vi "Sine Sweep Signal.vi"(0 "reference in":refnum<class "GSwFormDSP.lvclass">, 5 "error in (no error)":errorcluster) -> (14 "reference in":refnum<class "GSwFormDSP.lvclass">, 19 "error out":errorcluster)   [LabVIEW 2020, in "GSwFormDSP.lvclass"]
uses:
  GSwFormDSP.lvclass
panel:
  out "FS":dbl
  in  "Done":bool
  in  "Duration (s)":dbl=10.0 min=1.0 max=3600.0 step=0.1 format="%.1f"
  in  "User Input Fs":T1(ring)=enum."44100 Hz" caption="Sampling Rate"
  in  "Freq start (Hz)":dbl=100.0 min=0.0 max=22050.0 step=1.0 format="%.2f"
  in  "Freq end (Hz)":dbl=10000.0 min=0.0 max=22050.0 step=1.0 format="%.2f"
  in  "Amplitude":dbl=1.0 format="%.2f"
  in  "Signal Name":string="unknown"
  in  "Signal Unit":string="unknown"
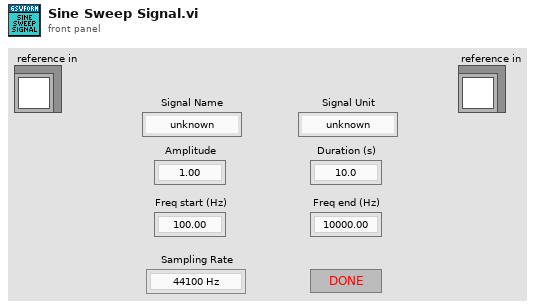
[diagram p1: front panel]
types:
  T1 = enum16{"256 Hz", "512 Hz", "1024 Hz", "2048 Hz", "4096 Hz", "8192 Hz", "11025 Hz", "16384 Hz", "22050 Hz", "32768 Hz", "44100 Hz"}
  T2 = enum16{"Replace Current Signals", "Append to Current Signals"}
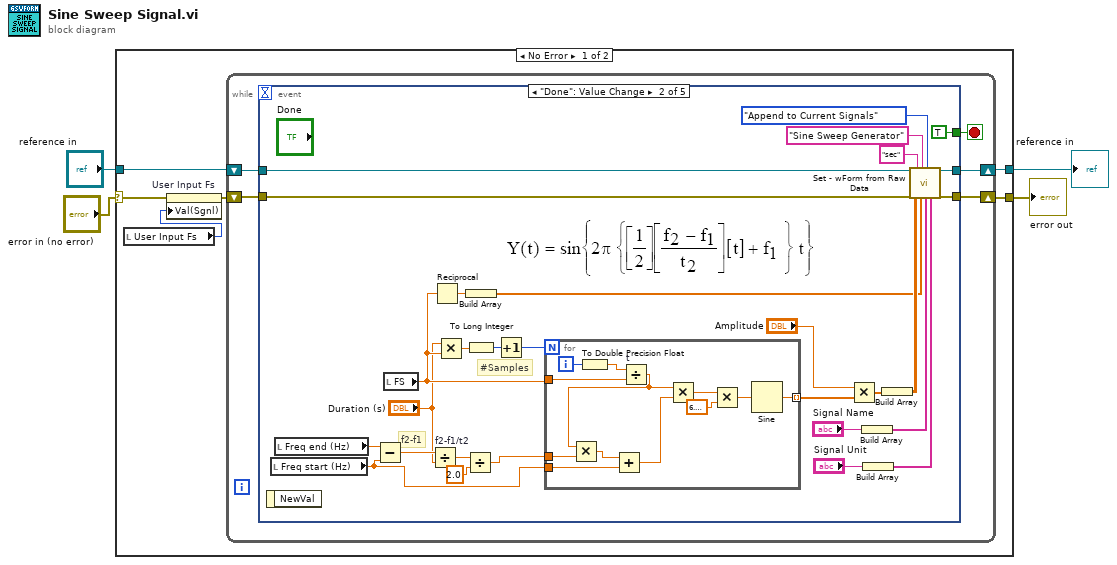
[diagram p0: block diagram]
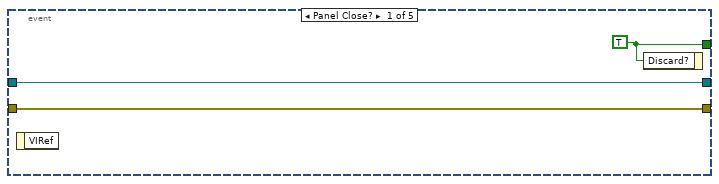
[diagram p2: hidden frame]
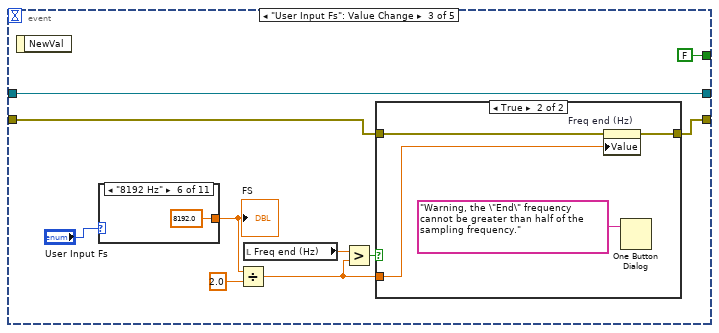
[diagram p3: hidden frame]
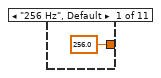
[diagram p5: hidden frame]
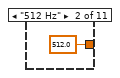
[diagram p6: hidden frame]
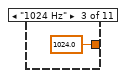
[diagram p7: hidden frame]
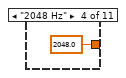
[diagram p8: hidden frame]
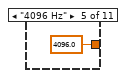
[diagram p9: hidden frame]
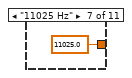
[diagram p10: hidden frame]
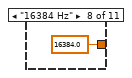
[diagram p11: hidden frame]
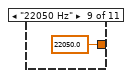
[diagram p12: hidden frame]
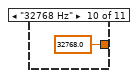
[diagram p13: hidden frame]
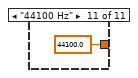
[diagram p14: hidden frame]
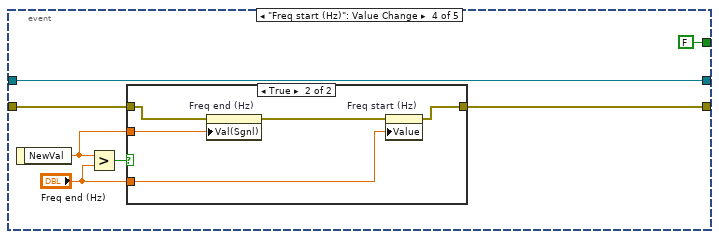
[diagram p15: hidden frame]
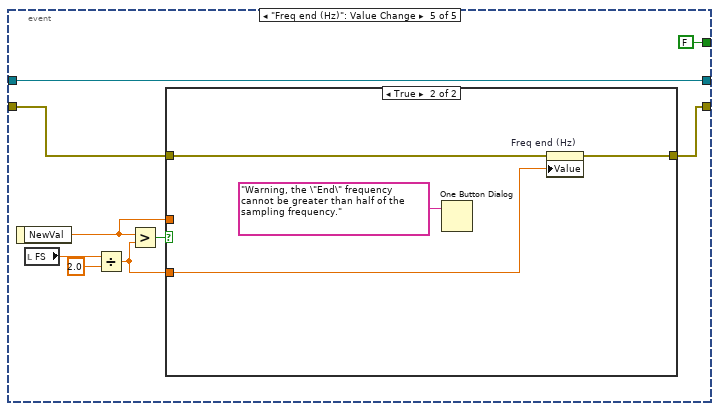
[diagram p17: hidden frame]
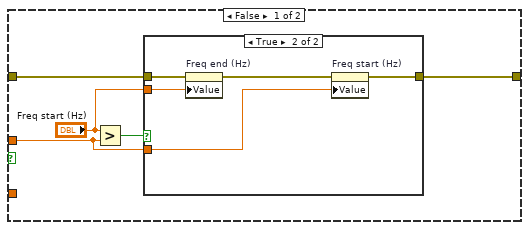
[diagram p18: hidden frame]
diagram:
  n1 = case shown="No Error" "error in (no error)" {
    selector: "error in (no error)" -> [w5 w124]
    tunnel: [w8 w124] -> w3
    tunnel: [w9 w123] -> w1
    tunnel: "reference in" -> [w10 w123]
    frame No Error {
      n2 = local read "User Input Fs"() -> (w6:T1)
      n3 = property on="User Input Fs" class="Enum (strict)"(error in=w5, "Val(Sgnl)"=w6) -> (error out=w7:errorcluster)  [unwired: 1 in, 1 out]
      n4 = while {
        shift-right: [w13] -> w9
        shift-left: w10 -> [w14]
        shift-right: [w12] -> w8
        shift-left: w7 -> [w11]
        stop <- w15 stop-if-true
        n5 = event shown="[1] \"Done\": Value Change" {
          selector: _ -> [_ _ _ _ _]
          dyn-events: _ -> [_ _ _ _ _]
          timeout: _ -> [_ _ _ _ _]
          tunnel: [w18 TRUE ("Discard?") FALSE ("Discard?") FALSE ("Discard?") FALSE ("Discard?")] -> w15
          tunnel: w14 -> [w17 w24 w67 w91 w106]
          tunnel: [w17 w23 w67 w91 w106] -> w13
          tunnel: [w16 w22 w61 w86 w102] -> w12
          tunnel: w11 -> [w16 w21 w62 w89 w103]
          event Panel Close? {
            w18 = TRUE ("Discard?")
            n6 = event-data() -> ()  [unwired: 1 in, 1 out]
            n7 = event-data("Discard?"=w18) -> ()  [unwired: 1 in, 1 out]
          }
          event "Done": Value Change {
            # "#Samples"
            # "f2-f1"
            n8 = event-data() -> ()  [unwired: 1 in, 1 out]
            n9 = local read "Freq start (Hz)"() -> (w28:dbl)
            n10 = local read "Freq end (Hz)"() -> (w29:dbl)
            n11 = Subtract(x=w29, y=w28) -> (x-y=w45:dbl)
            n12 = local read "FS"() -> (w30:dbl)
            n13 = Divide "f2-f1/t2"(x=w45, y="Duration (s)") -> (x/y=w42:dbl)
            n14 = Reciprocal(x=w30) -> (1/x=w38:dbl)
            n15 = Multiply(x="Duration (s)", y=w30) -> (x*y=w46:dbl)
            n16 = Divide(x=w42, y=2.0) -> (x/y=w40:dbl)
            n17 = Build Array(w38) -> (w34:dbl[])
            n18 = To Long Integer(number=w46) -> (32bit integer=w41:i32)
            n19 = Increment(x=w41) -> (x+1=w43:i32)
            n20 = for {
              N: w43 -> [_]
              tunnel: [w57] -> w44 mode=indexing
              tunnel: w40 -> [w56]
              tunnel: w28 -> [w54]
              tunnel: w30 -> [w53]
              i -> [w50]
              n21 = To Double Precision Float(number=w50) -> (double precision float=w49:dbl)
              n22 = Divide "t"(x=w49, y=w53) -> (x/y=w48:dbl)
              n23 = Multiply(x=w48, y=w56) -> (x*y=w55:dbl)
              n24 = Add(x=w55, y=w54) -> (x+y=w51:dbl)
              n25 = Multiply(x=w48, y=w51) -> (x*y=w52:dbl)
              n26 = Multiply(x=w52, y=6.283185307179586) -> (x*y=w59:dbl)
              n27 = Sine(x=w59) -> (sin(x)=w57:dbl)
            }
            n28 = Multiply(x="Amplitude", y=w44) -> (x*y=w27:dbl[])
            n29 = Build Array("Signal Name") -> (w33:string[])
            n30 = Build Array("Signal Unit") -> (w32:string[])
            n31 = Build Array(w27) -> (w35:dbl[][])
            n32 = call "Set - wForm from Raw Data.vi"("reference in"=w24, "error in (no error)"=w21, "X Unit"="sec", "Y Data (Row matrix)"=w35, "Data Origin"="Sine Sweep Generator", "dTs"=w34, "Signal Set"=T2."Append to Current Signals", "Signals Name"=w33, "Signals Unit"=w32) -> ("reference in"=w23:refnum<class "GSwFormDSP.lvclass">, "error out"=w22:errorcluster)  [unwired: 9 in]
          }
          event "User Input Fs": Value Change {
            n33 = event-data() -> ()  [unwired: 1 in, 1 out]
            n34 = case shown="\"8192 Hz\"" "User Input Fs" {
              tunnel: [256.0 512.0 1024.0 2048.0 4096.0 8192.0 11025.0 16384.0 22050.0 32768.0 44100.0] -> w65
              frame "256 Hz", Default {
              }
              frame "512 Hz" {
              }
              frame "1024 Hz" {
              }
              frame "2048 Hz" {
              }
              frame "4096 Hz" {
              }
              frame "8192 Hz" {
              }
              frame "11025 Hz" {
              }
              frame "16384 Hz" {
              }
              frame "22050 Hz" {
              }
              frame "32768 Hz" {
              }
              frame "44100 Hz" {
              }
            }
            "FS" <- w65
            n35 = Divide(x=w65, y=2.0) -> (x/y=w60:dbl)
            n36 = local read "Freq end (Hz)"() -> (w64:dbl)
            n37 = Greater?(x=w64, y=w60) -> (0:w63:bool)
            n38 = case shown="True" w63 {
              tunnel: w62 -> [w70 w73]
              tunnel: [w70 w72] -> w61
              tunnel: w60 -> [_ w71]
              frame False {
              }
              frame True {
                n39 = property on="Freq end (Hz)" class="DigNum (strict)"(error in=w73, "Value"=w71) -> (error out=w72:errorcluster)  [unwired: 1 in, 1 out]
                n40 = One Button Dialog(message="Warning, the \"End\" frequency cannot be greater than half of the sampling frequency.") -> ()  [unwired: 1 in, 1 out]
              }
            }
          }
          event "Freq start (Hz)": Value Change {
            n41 = event-data() -> ("NewVal"=w88:dbl)  [unwired: 1 in]
            n42 = Greater?(x=w88, y="Freq end (Hz)") -> (0:w90:bool)
            n43 = case shown="True" w90 {
              tunnel: w89 -> [w93 w98]
              tunnel: w88 -> [_ w97]
              tunnel: "Freq end (Hz)" -> [_ w96]
              tunnel: [w93 w94] -> w86
              frame False {
              }
              frame True {
                n44 = property on="Freq end (Hz)" class="DigNum (strict)"(error in=w98, "Val(Sgnl)"=w97) -> (error out=w95:errorcluster)  [unwired: 1 in, 1 out]
                n45 = property on="Freq start (Hz)" class="DigNum (strict)"(error in=w95, "Value"=w96) -> (error out=w94:errorcluster)  [unwired: 1 in, 1 out]
              }
            }
          }
          event "Freq end (Hz)": Value Change {
            n46 = event-data() -> ("NewVal"=w104:dbl)  [unwired: 1 in]
            n47 = local read "FS"() -> (w100:dbl)
            n48 = Divide(x=w100, y=2.0) -> (x/y=w99:dbl)
            n49 = Greater?(x=w104, y=w99) -> (0:w105:bool)
            n50 = case shown="True" w105 {
              tunnel: w104 -> [w110 _]
              tunnel: w103 -> [w109 w121]
              tunnel: [w108 w120] -> w102
              tunnel: w99 -> [_ w119]
              frame False {
                n51 = Greater?(x="Freq start (Hz)", y=w110) -> (0:w112:bool)
                n52 = case shown="True" w112 {
                  tunnel: "Freq start (Hz)" -> [_ w118]
                  tunnel: w110 -> [_ w117]
                  tunnel: w109 -> [w113 w115]
                  tunnel: [w113 w114] -> w108
                  frame False {
                  }
                  frame True {
                    n53 = property on="Freq end (Hz)" class="DigNum (strict)"(error in=w115, "Value"=w118) -> (error out=w116:errorcluster)  [unwired: 1 in, 1 out]
                    n54 = property on="Freq start (Hz)" class="DigNum (strict)"(error in=w116, "Value"=w117) -> (error out=w114:errorcluster)  [unwired: 1 in, 1 out]
                  }
                }
              }
              frame True {
                n55 = One Button Dialog(message="Warning, the \"End\" frequency cannot be greater than half of the sampling frequency.") -> ()  [unwired: 1 in, 1 out]
                n56 = property on="Freq end (Hz)" class="DigNum (strict)"(error in=w121, "Value"=w119) -> (error out=w120:errorcluster)  [unwired: 1 in, 1 out]
              }
            }
          }
        }
      }
    }
    frame Error {
    }
  }
  "error out" <- w3
  "reference in" <- w1
